vi "Tile Plot.vi"() -> ()   [LabVIEW 2011]
uses:
  <vilib>/Heliosphere Research LLC/Advanced Plotting Toolkit/Advanced Plotting Toolkit.lvlib
  <vilib>/Heliosphere Research LLC/Advanced Plotting Toolkit/properties/Colormap_Map.ctl
  <vilib>/Heliosphere Research LLC/Advanced Plotting Toolkit/properties/Colormap_Scaling.ctl
  <vilib>/Heliosphere Research LLC/Advanced Plotting Toolkit/properties/Colormap.ctl
  <vilib>/Heliosphere Research LLC/Advanced Plotting Toolkit/properties/Line_Style.ctl
  <vilib>/Heliosphere Research LLC/Advanced Plotting Toolkit/typedefs/PlotColor.ctl
  <vilib>/Heliosphere Research LLC/Advanced Plotting Toolkit/properties/Line.ctl
  <vilib>/Heliosphere Research LLC/Advanced Plotting Toolkit/properties/Display.ctl
  <vilib>/Heliosphere Research LLC/Advanced Plotting Toolkit/api_plotting/TilesProperties.ctl
panel:
  in  "Line Width":sgl=nan
  in  "Line Color":T1=2147483647 items=["Automatic"=2147483647, "Black"=0, "White"=16777215, "Red"=16711680, "Green"=2263842, "Blue"=255, "Cyan"=65535, "Magenta"=16711935, "Yellow"=16776960]
  in  "Colormap":T2
  out "Tile Plot":picture
  # "Tiles"
  # "This VI demonstrates a \"tile\" plot, in which the elements of an\narray are displayed as colored rectangles.  These plots are\nsimilar in appearance to 2D histogram plots, but are not limited\nto displaying histogram data.\n\nSupply a 2D array and (optionally) X and Y arrays giving the\nlocation of lines at the tile boundaries.  You can also choose\nthe colormap used to display the tiles, and change the\nappearance of the lines between tiles.\n\nTry changing the Line Color to \"White\", below."
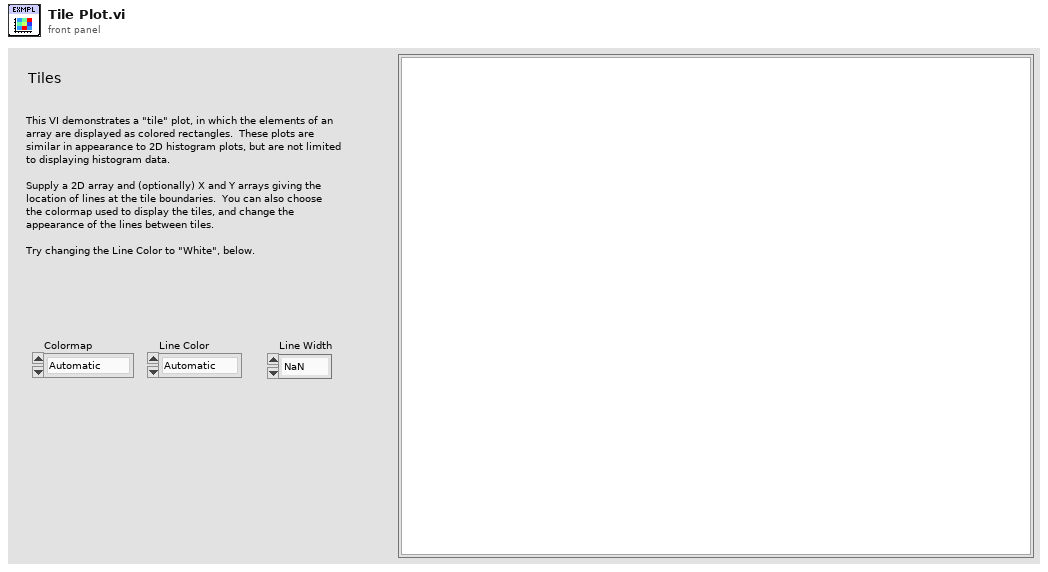
[diagram p1: front panel]
types:
  T1 = typedef "Advanced Plotting Toolkit.lvlib/PlotColor.ctl" = u32
  T2 = typedef "Advanced Plotting Toolkit.lvlib/Colormap_Map.ctl" = enum16{"Automatic", "Rainbow", "Hot and Cold", "White-Black", "White-Blue", "White-Green", "White-Red", "Fire", "Water", "Earth", "Air", "Pastel", "Banded", "Stepped"}
  T3 = typedef "Advanced Plotting Toolkit.lvlib/TilesProperties.ctl" = cluster{"Colormap":T4, "Line":T6, "Display":T8}
  T4 = typedef "Advanced Plotting Toolkit.lvlib/Colormap.ctl" = cluster{"Map":T2, "Value Min":dbl, "Value Max":dbl, "Scaling":T5, "Reverse":bool}
  T5 = typedef "Advanced Plotting Toolkit.lvlib/Colormap_Scaling.ctl" = enum16{"Default"}
  T6 = typedef "Advanced Plotting Toolkit.lvlib/Line.ctl" = cluster{"Style":T7, "Color":T1, "Width":sgl}
  T7 = typedef "Advanced Plotting Toolkit.lvlib/Line_Style.ctl" = enum16{"Automatic", "Solid", "Dashed", "Dotted", "Dash-dot", "Invisible"}
  T8 = typedef "Advanced Plotting Toolkit.lvlib/Display.ctl" = cluster{"Alpha":dbl, "Z Order":dbl}
  T9 = typedef "Advanced Plotting Toolkit.lvlib/PlotID.ctl" = i32
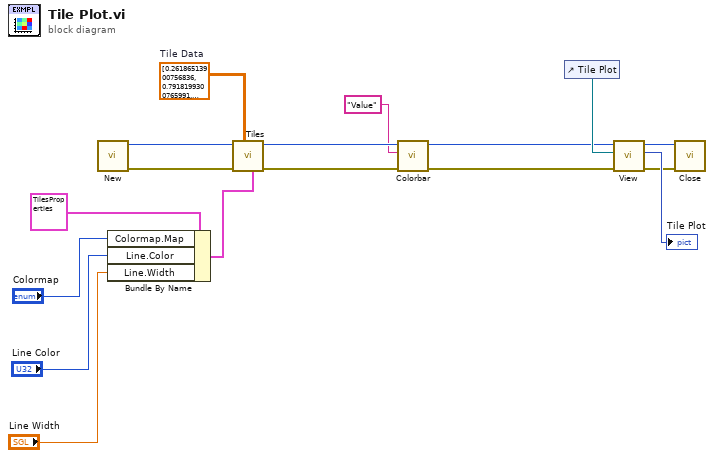
[diagram p0: block diagram]
diagram:
  w12 = sgl[][] [[0.26186514, 0.79181993, 0.6813736, 0.9868132, 0.3343468, 0.2647247, 0.8865877, 0.8101756, 0.084153175, 0.18005297], [0.5078847, 0.19216605, 0.45872653, 0.59001005, 0.09002146, 0.08245192, 0.21045662, 0.862694, 0.30868667, 0.1349976], [0.402347, 0.5071572, 0.35049453, 0.76479155, 0.7870985, 0.22492626, 0.71743107, 0.21907695, 0.49101835, 0.7285668], [0.3684696, 0.8566974, 0.40341404, 0.18016115, 0.3284572, 0.46725088, 0.7992155, 0.70721537, 0.57653797, 0.20412567], [0.5373711, 0.86141026, 0.28710404, 0.10478162, 0.8900068, 0.8505361, 0.7807401, 0.27852455, 0.05683467, 0.48206082], [0.791165, 0.27637172, 0.5239455, 0.43708882, 0.3449234, 0.95939934, 0.63072664, 0.037709404, 0.9607076, 0.9349509], [0.027474342, 0.9974626, 0.24009068, 0.25674808, 0.6657562, 0.10189452, 0.4339676, 0.42299813, 0.62083375, 0.92179996], [0.1487872, 0.7398255, 0.52051735, 0.74713457, 0.8420234, 0.443048, 0.25370622, 0.73401535, 0.059708044, 0.06999489], [0.3825536, 0.5047975, 0.3694082, 0.938698, 0.0016683866, 0.82069117, 0.48330888, 0.97105205, 0.20352715, 0.112183206], [0.2587809, 0.8201253, 0.6770269, 0.85123974, 0.23831576, 0.11277079, 0.4649663, 0.82599306, 0.86109364, 0.0104329]]  # Tile Data
  n1 = call <vilib>:"New.vi"() -> ("error out"=w13:errorcluster, "Plot ID"=w14:T9)  [unwired: 10 in]
  n2 = Bundle By Name(cluster=T3 {"Colormap"={"Map"=enum."Automatic", "Value Min"=nan, "Value Max"=nan, "Scaling"=enum."Default", "Reverse"=FALSE}, "Line"={"Style"=enum."Automatic", "Color"=2147483647, "Width"=nan}, "Display"={"Alpha"=nan, "Z Order"=nan}} ("Properties"), "Colormap.Map"="Colormap", "Line.Color"="Line Color", "Line.Width"="Line Width") -> (w10:T3)
  n3 = call <vilib>:"Tiles.vi"("Properties"=w10, "Z Data"=w12, "error in (no error)"=w13, "Plot ID"=w14) -> ("error out"=w5:errorcluster, "Plot ID Out"=w8:T9)  [unwired: 6 in]
  n4 = call <vilib>:"Colorbar.vi"("error in (no error)"=w5, "Label"="Value", "Plot ID"=w8) -> ("error out"=w6:errorcluster, "Plot ID Out"=w7:T9)  [unwired: 7 in]
  n5 = control-ref of="Tile Plot"() -> (w16:refnum<vi>)
  n6 = call <vilib>:"View.vi"("error in (no error)"=w6, "Ref for Sizing"=w16, "Plot ID"=w7) -> ("error out"=w1:errorcluster, "Picture"=→"Tile Plot":picture, "Plot ID Out"=w15:T9)  [unwired: 6 in]
  n7 = call <vilib>:"Close.vi"("error in (no error)"=w1, "Plot ID"=w15) -> ()  [unwired: 9 in, 1 out]
